vi "read mapping data.vi"(8 "error in (no error)":errorcluster, 11 "BMC in":refnum<class "BMC.lvclass">) -> (0 "error out":errorcluster, 3 "BMC out":refnum<class "BMC.lvclass">)   [LabVIEW 2012, in "BMC.lvclass"]
uses:
  BMC.lvclass
  BMC.lvclass/BMC.ctl
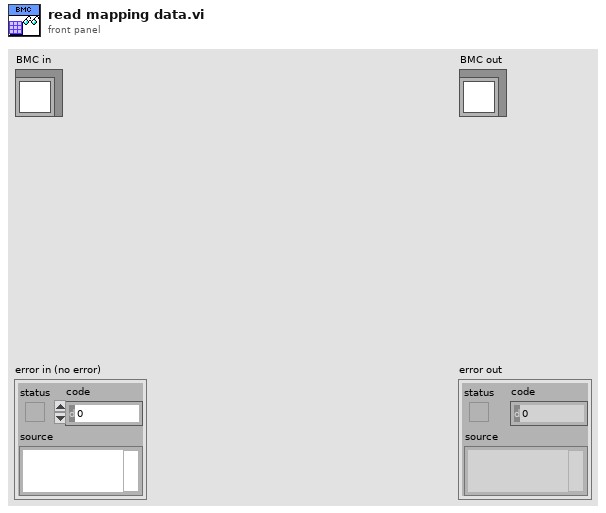
[diagram p1: front panel]
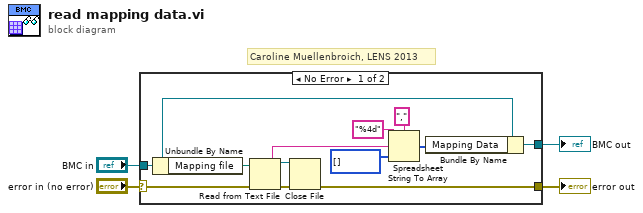
[diagram p0: block diagram]
diagram:
  # "Caroline Muellenbroich, LENS 2013"
  n1 = case shown="No Error" "error in (no error)" {
    selector: "error in (no error)" -> [w11 w18]
    tunnel: [w10 w18] -> w3
    tunnel: "BMC in" -> [w9 w17]
    tunnel: [w8 w17] -> w1
    frame No Error {
      n2 = Unbundle By Name(w9) -> ("Mapping file"=w5:path)
      n3 = Read from Text File(file (use dialog)=w5, error in=w11) -> (refnum out=w15:refnum<file>, text=w12:string, error out=w16:errorcluster)  [unwired: 3 out]
      n4 = Close File(refnum=w15, error in=w16) -> (error out=w10:errorcluster)  [unwired: 1 out]
      n5 = Spreadsheet String To Array(delimiter (Tab)=",", format string="%4d", spreadsheet string=w12, array type (2D Dbl)=i32[] [] ("run time Cluster.Mapping Data")) -> (array=w6:i32[])
      n6 = Bundle By Name(cluster=w9, "Mapping Data"=w6) -> (w8:refnum<class "BMC.lvclass">)
    }
    frame Error {
    }
  }
  "error out" <- w3
  "BMC out" <- w1
